vi "Graphics.vi"() -> ()   [LabVIEW 2023]
doc: "This example demonstrates a traditional hierarchy of classes. The Line, Point, and Collection\nclasses inherit from the Graphic class."
uses:
  Line/Line example.lvclass
  c:/dev/_r/4/eng/lv-core/lvpostprocessingd/lv_mc_x86_64/dist_i386/examples/Object-Oriented Programming/Graphics/Graphic/Graphic.lvclass
  Collection/Collection.lvclass
  Circle/Circle.lvclass
  Point/Point.lvclass
  Graphic/Graphic.lvclass
panel:
  in  "Center Y":i16=150
  in  "Center X":i16=50
  in  "Inner Circle Color":u32(colorbox)=16777215
  in  "Outer Circle Color":u32(colorbox)=14423296
  in  "Outer Radius":u16=10
  in  "Line Color":u32(colorbox)=786687
  in  "Y 3":i16=150
  in  "X 3":i16=50
  in  "Y 2":i16=150
  in  "X 2":i16=250
  in  "Y":i16=50
  in  "X":i16=150
  out "Picture":picture
  # "Overview: Demonstrates a traditional hierarchy of classes. The Line, Point, Circle and Collection classes inherit from the Graphic class.\nInstructions:\n1. Set the three points for a triangle: (X, Y), (X 2, Y 2) and (X3, Y3). \n2. Run the VI.\n3. Open the block diagram and refer to the comments."
  # "Line Options"
  # "Circle Options"
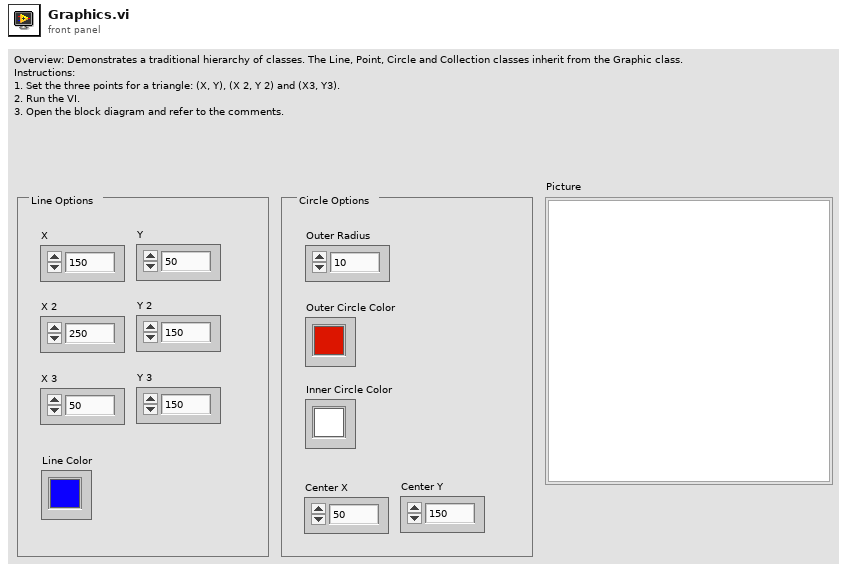
[diagram p1: front panel]
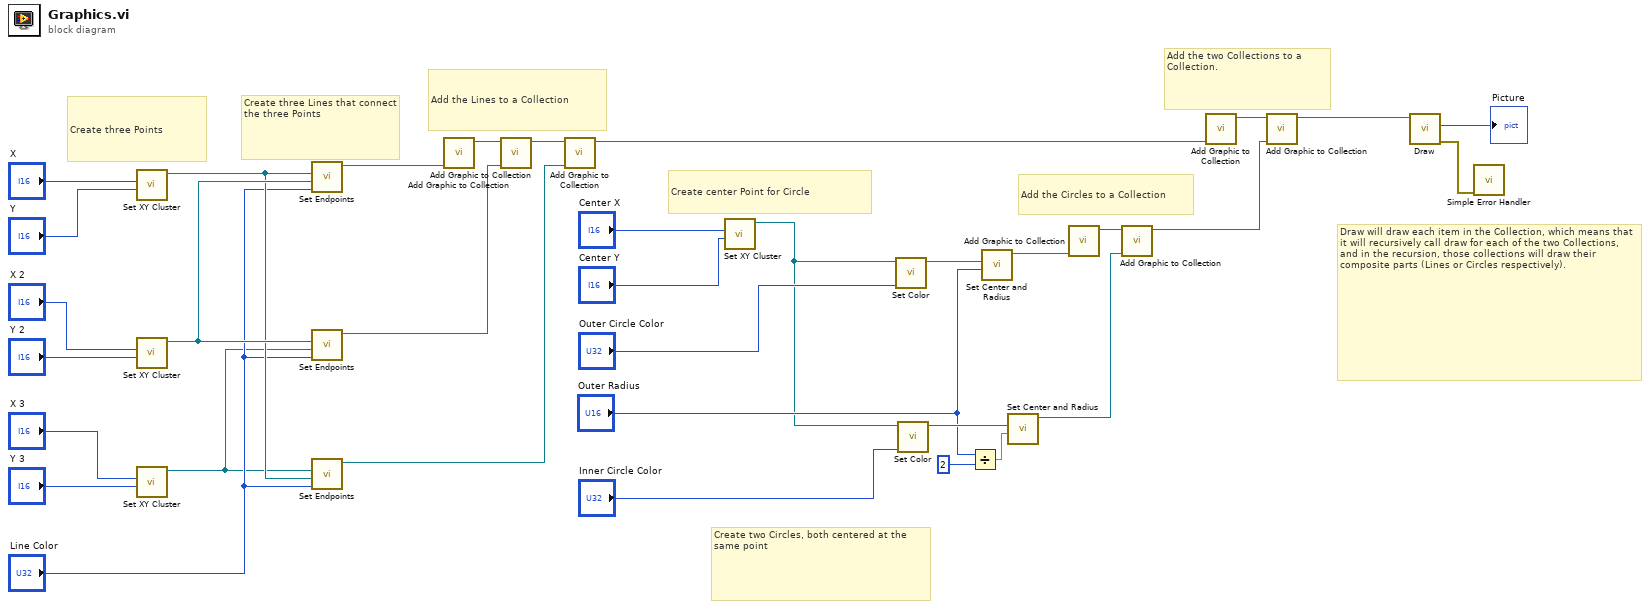
[diagram p0: block diagram]
diagram:
  # "Create center Point for Circle"
  # "Add the two Collections to a Collection."
  # "Create three Points"
  # "Draw will draw each item in the Collection, which means that it will recursively call draw for each of the two Collections, and in the recursion, those collections will draw their composite parts (Lines or Circles respectively)."
  # "Add the Circles to a Collection"
  # "Add the Lines to a Collection"
  # "Create three Lines that connect the three Points"
  # "Create two Circles, both centered at the same point"
  n1 = call "Set XY Cluster.vi"("Y"="Y", "X"="X") -> ("Point Out"=w26:refnum<class "Point.lvclass">)  [unwired: 2 in, 7 out]
  n2 = call "Set XY Cluster.vi"("Y"="Y 2", "X"="X 2") -> ("Point Out"=w27:refnum<class "Point.lvclass">)  [unwired: 2 in, 7 out]
  n3 = call "Set XY Cluster.vi"("Y"="Y 3", "X"="X 3") -> ("Point Out"=w11:refnum<class "Point.lvclass">)  [unwired: 2 in, 7 out]
  n4 = call "Set Endpoints.vi"("Color"="Line Color", "B"=w27, "A"=w26) -> ("Line out"=w30:refnum<class "Line example.lvclass">)  [unwired: 1 in, 7 out]
  n5 = call "Set Endpoints.vi"("Color"="Line Color", "B"=w11, "A"=w27) -> ("Line out"=w22:refnum<class "Line example.lvclass">)  [unwired: 1 in, 7 out]
  n6 = call "Set Endpoints.vi"("Color"="Line Color", "B"=w26, "A"=w11) -> ("Line out"=w21:refnum<class "Line example.lvclass">)  [unwired: 1 in, 7 out]
  n7 = call "Add Graphic to Collection.vi"("Graphic"=w30) -> ("Collection of Graphics Out"=w24:refnum<class "Collection.lvclass">)  [unwired: 1 in, 9 out]
  n8 = call "Add Graphic to Collection.vi"("Graphic"=w22, "Collection of Graphics In"=w24) -> ("Collection of Graphics Out"=w23:refnum<class "Collection.lvclass">)  [unwired: 9 out]
  n9 = call "Add Graphic to Collection.vi"("Graphic"=w21, "Collection of Graphics In"=w23) -> ("Collection of Graphics Out"=w20:refnum<class "Collection.lvclass">)  [unwired: 9 out]
  n10 = call "Set XY Cluster.vi"("Y"="Center Y", "X"="Center X") -> ("Point Out"=w4:refnum<class "Point.lvclass">)  [unwired: 2 in, 7 out]
  n11 = call "Set Color.vi"("Color"="Outer Circle Color", "Point In"=w4) -> ("Point Out"=w18:refnum<class "Point.lvclass">)  [unwired: 9 out]
  n12 = call "Set Color.vi"("Color"="Inner Circle Color", "Point In"=w4) -> ("Point Out"=w15:refnum<class "Point.lvclass">)  [unwired: 9 out]
  n13 = Divide(x="Outer Radius", y=u16 2 ("divide")) -> (x/y=w14:dbl)
  n14 = call "Set Center and Radius.vi"("Radius"="Outer Radius", "Point.lvclass"=w18) -> ("Circle out"=w8:refnum<class "Circle.lvclass">)  [unwired: 1 in, 8 out]
  n15 = call "Set Center and Radius.vi"("Radius"=w14, "Point.lvclass"=w15) -> ("Circle out"=w9:refnum<class "Circle.lvclass">)  [unwired: 1 in, 8 out]
  n16 = call "Add Graphic to Collection.vi"("Graphic"=w8) -> ("Collection of Graphics Out"=w10:refnum<class "Collection.lvclass">)  [unwired: 1 in, 9 out]
  n17 = call "Add Graphic to Collection.vi"("Graphic"=w9, "Collection of Graphics In"=w10) -> ("Collection of Graphics Out"=w7:refnum<class "Collection.lvclass">)  [unwired: 9 out]
  n18 = call "Add Graphic to Collection.vi"("Graphic"=w20) -> ("Collection of Graphics Out"=w19:refnum<class "Collection.lvclass">)  [unwired: 1 in, 9 out]
  n19 = call "Add Graphic to Collection.vi"("Graphic"=w7, "Collection of Graphics In"=w19) -> ("Collection of Graphics Out"=w17:refnum<class "Collection.lvclass">)  [unwired: 9 out]
  n20 = call "Draw.vi"("Graphic In"=w17) -> ("error out"=w1:errorcluster, "Picture out"=→"Picture":picture)  [unwired: 2 in, 7 out]
  n21 = call <vilib>:"Simple Error Handler.vi"("error in (no error)"=w1) -> ()  [unwired: 4 in, 5 out]
